vi "Test Image Creation.vi"(8 "error in (no error)":errorcluster, 11 "Test Case In":refnum<class "Image.lvclass">) -> (0 "error out":errorcluster, 3 "Test Case Out":refnum<class "Image.lvclass">)   [LabVIEW 2020, in "g_ar_toolkit.test.lvlib" / "Image.lvclass"]
uses:
  Image.lvclass
  Image.lvclass/Image.ctl
  g_ar_toolkit.image/g_ar_toolkit.image.lvlib
  g_ar_toolkit.image/CreateEmptyImageARGB.vi
  g_ar_toolkit.image/CreateEmptyImageGreyscale.vi
  g_ar_toolkit.common/Image Size (Integer).ctl
  g_ar_toolkit.common/g_ar_toolkit.common.lvlib
  0bcaab8e-db39-49f4-b03c-e96854e28b99.vi
  ec21ac67-ee19-4f7a-8949-2d8c4815d422.vi
  4247fbd1-0910-49f6-b629-9f858556f783.vi
  ef19801d-c7eb-448b-804c-03b939946be6.vi
  g_ar_toolkit.image/ARGB Colour.ctl
  a2513b5f-71c0-4474-9565-80dd8f5665c2.vi
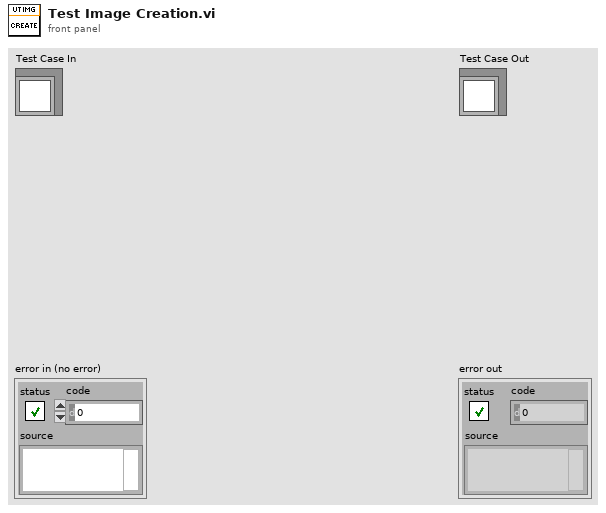
[diagram p1: front panel]
types:
  T1 = enum16{"ARGB empty", "Greyscale empty", "ARGB with size", "Greyscale with size"}
  T2 = typedef "g_ar_toolkit.common.lvlib/Image Size (Integer).ctl" = cluster{"Width":u16, "Height":u16}
  T3 = enum16{"ARGB empty", "Greyscale empty", "ARGB with size", "Greyscale with size"}[]
  T4 = typedef "g_ar_toolkit.image.lvlib/ARGB Colour.ctl" = cluster{"Alpha":u8, "RGB":u32}
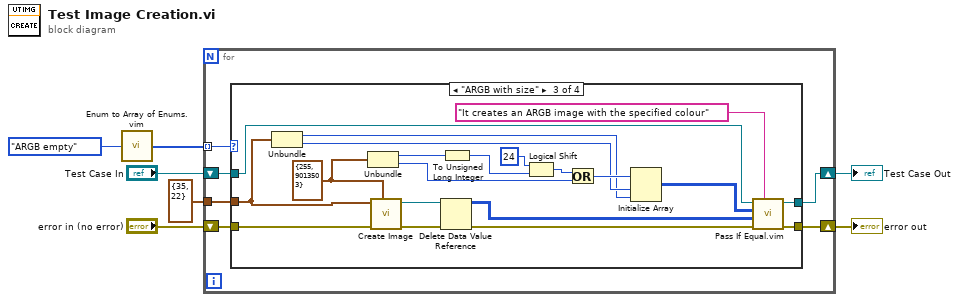
[diagram p0: block diagram]
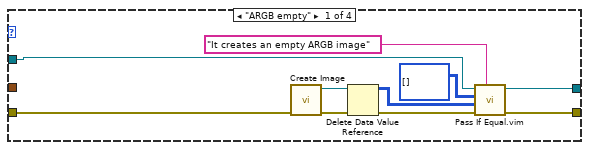
[diagram p2: hidden frame]
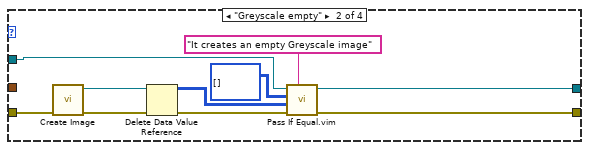
[diagram p3: hidden frame]
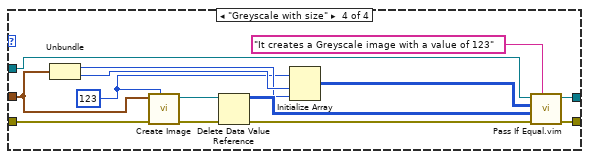
[diagram p4: hidden frame]
diagram:
  n1 = call "Enum to Array of Enums.vim"("enum"=T1."ARGB empty") -> ("array of enums"=w2:T3)
  n2 = for {
    shift-right: [w10] -> w6
    shift-left: "Test Case In" -> [w13]
    shift-right: [w9] -> w4
    shift-left: "error in (no error)" -> [w12]
    tunnel: w2 -> [w11] mode=indexing
    tunnel: T2 {"Width"=35, "Height"=22} ("Preallocated Image Size (Default: 0,0)") -> [w8]
    n3 = case shown="\"ARGB with size\"" w11 {
      tunnel: w13 -> [w17 w30 w47 w61]
      tunnel: w12 -> [w23 w33 w53 w67]
      tunnel: [w18 w29 w48 w62] -> w10
      tunnel: [w19 w27 w49 w63] -> w9
      tunnel: w8 -> [_ _ w37 w58]
      frame "ARGB empty" {
        n4 = call-poly "Create Image.vi"("error in (no error)"=w23) -> ("error out"=w22:errorcluster, "New ARGB Image"=w21:refnum<data-value>)  [unwired: 9 in]
        n5 = Delete Data Value Reference(data value reference=w21, error in=w22) -> (data value=w16:u32[][], error out=w20:errorcluster)
        n6 = call "Pass If Equal.vim"("Description"="It creates an empty ARGB image", "error in (no error)"=w20, "Actual"=w16, "Expected"=u32[][] [] ("data value"), "LUnit Test Case In"=w17) -> ("error out"=w19:errorcluster, "LUnit Test Case Out"=w18:refnum<class "Image.lvclass">)  [unwired: 5 in]
      }
      frame "Greyscale empty" {
        n7 = call-poly "Create Image.vi"("error in (no error)"=w33) -> ("error out"=w32:errorcluster, "New Greyscale Image"=w31:refnum<data-value>)  [unwired: 9 in]
        n8 = Delete Data Value Reference(data value reference=w31, error in=w32) -> (data value=w25:u8[][], error out=w28:errorcluster)
        n9 = call "Pass If Equal.vim"("Description"="It creates an empty Greyscale image", "error in (no error)"=w28, "Actual"=w25, "Expected"=u8[][] [] ("data value"), "LUnit Test Case In"=w30) -> ("error out"=w27:errorcluster, "LUnit Test Case Out"=w29:refnum<class "Image.lvclass">)  [unwired: 5 in]
      }
      frame "ARGB with size" {
        w44 = T4 {"Alpha"=255, "RGB"=9013503} ("Colour (Default: Black)")
        n10 = Unbundle(w37) -> ("Width"=w35:u16, "Height"=w36:u16)
        n11 = Unbundle(w44) -> ("Alpha"=w42:u8, "RGB"=w43:u32)
        n12 = call-poly "Create Image.vi"("Colour (Default: Black)"=w44, "error in (no error)"=w53, "Preallocated Image Size (Default: 0,0)"=w37) -> ("error out"=w52:errorcluster, "New ARGB Image"=w51:refnum<data-value>)  [unwired: 7 in]
        n13 = Delete Data Value Reference(data value reference=w51, error in=w52) -> (data value=w46:u32[][], error out=w50:errorcluster)
        n14 = To Unsigned Long Integer(number=w42) -> (unsigned 32bit integer=w41:u32)
        n15 = Logical Shift(y=i16 24, x=w41) -> (x << y=w40:u32)
        n16 = Or(x=w40, y=w43) -> (x .or. y?=w38:u32)
        n17 = Initialize Array(w38, w36, w35) -> (w34:u32[][])
        n18 = call "Pass If Equal.vim"("Description"="It creates an ARGB image with the specified colour", "error in (no error)"=w50, "Actual"=w46, "Expected"=w34, "LUnit Test Case In"=w47) -> ("error out"=w49:errorcluster, "LUnit Test Case Out"=w48:refnum<class "Image.lvclass">)  [unwired: 5 in]
      }
      frame "Greyscale with size" {
        w54 = u8 123 ("Value (Default: 0)")
        n19 = Unbundle(w58) -> ("Width"=w56:u16, "Height"=w57:u16)
        n20 = call-poly "Create Image.vi"("Value (Default: 0)"=w54, "error in (no error)"=w67, "Preallocated Image Size (Default 0,0)"=w58) -> ("error out"=w66:errorcluster, "New Greyscale Image"=w65:refnum<data-value>)  [unwired: 7 in]
        n21 = Delete Data Value Reference(data value reference=w65, error in=w66) -> (data value=w60:u8[][], error out=w64:errorcluster)
        n22 = Initialize Array(w54, w57, w56) -> (w55:u8[][])
        n23 = call "Pass If Equal.vim"("Description"="It creates a Greyscale image with a value of 123", "error in (no error)"=w64, "Actual"=w60, "Expected"=w55, "LUnit Test Case In"=w61) -> ("error out"=w63:errorcluster, "LUnit Test Case Out"=w62:refnum<class "Image.lvclass">)  [unwired: 5 in]
      }
    }
  }
  "error out" <- w4
  "Test Case Out" <- w6
